vi "Testing.vi"() -> ()   [LabVIEW 2024]
uses:
  <vilib>/Instr/_visa.llb/VISA Configure Serial Port (Instr).vi
panel:
  out "FrequencyCounter":refnum<visa-resource-name>
  out "connection information":path
  in  "Database Checker":bool
  in  "Test Type":u16(ring)=1 items=["FVT/OSC/PHN", "FVT/OSC", "FVT/PHN", "OSC/PHN", "FVT", "OSC", "PHN", "Warmup", "Output Powers", "Warmup/Output Powers"]
  out "TITLE":string
  out "System Number":string
  in  "Functional Test":bool
  out "Functional Test Data":string
  out "Time":string
  out "System Status":string
  in  "Run Test(s)":bool
  in  "Exit":bool
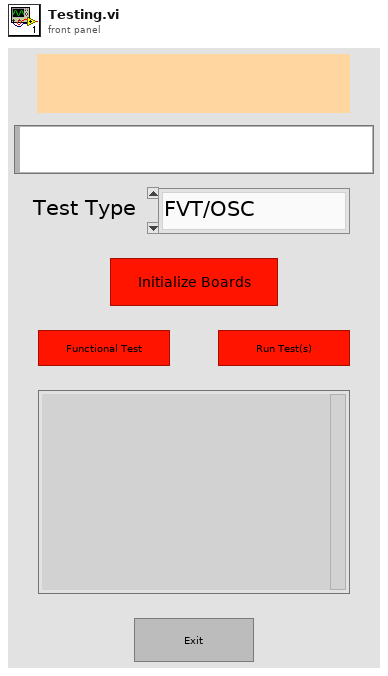
[diagram p1: front panel]
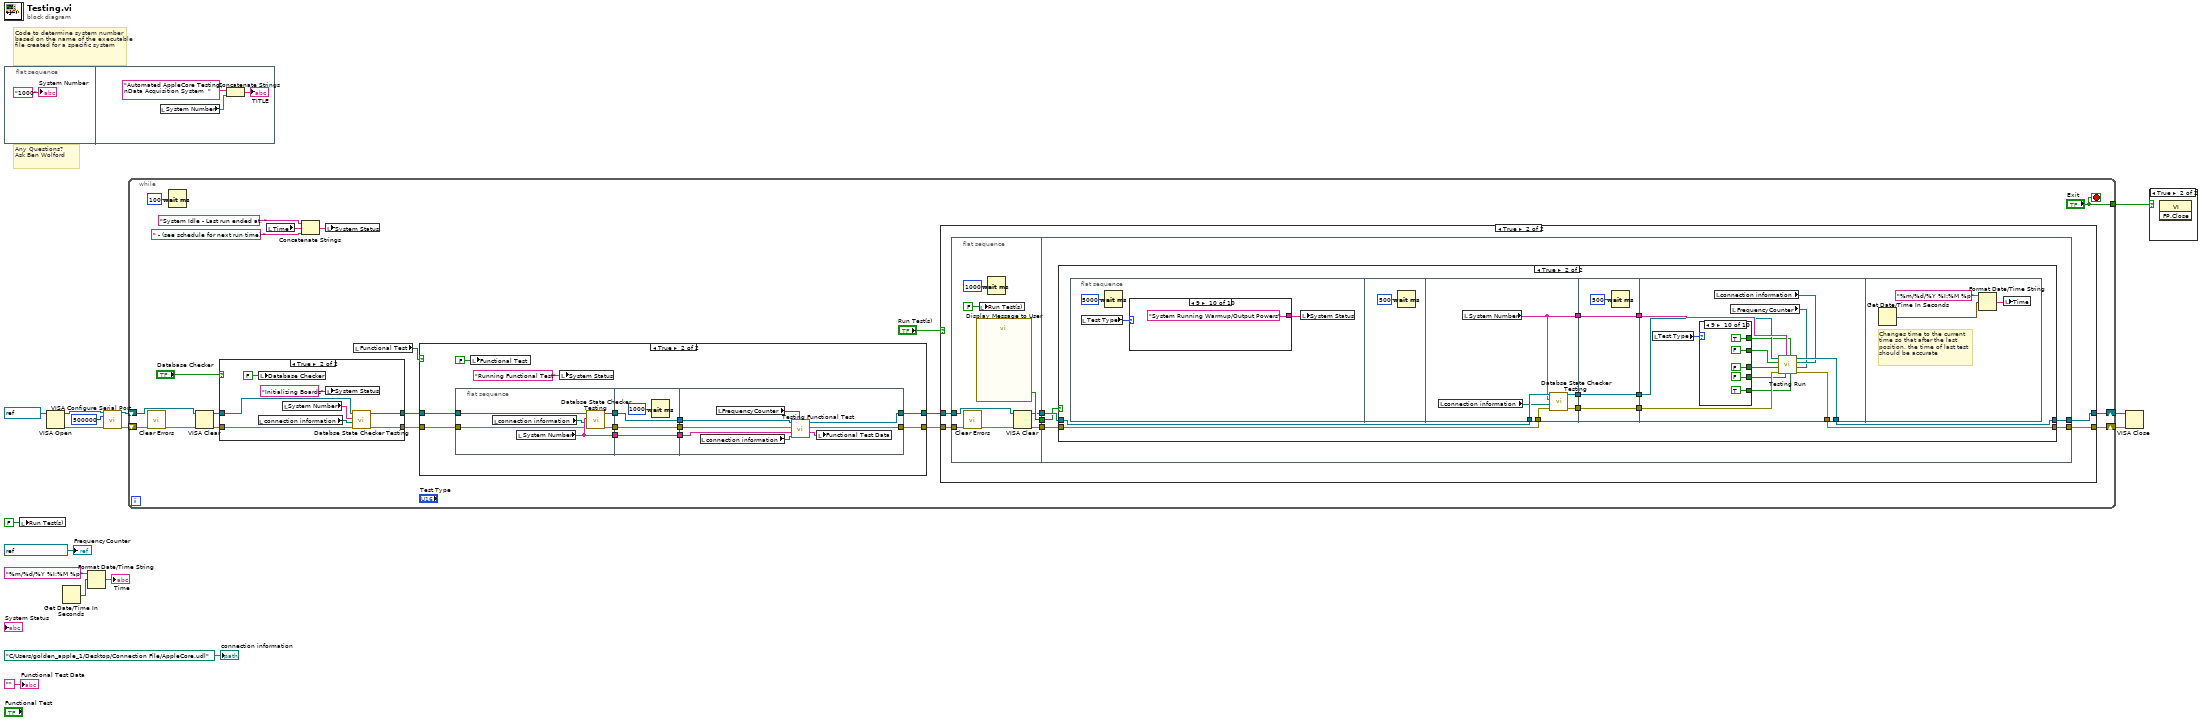
[diagram p0: block diagram]
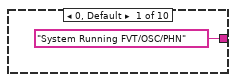
[diagram p7: hidden frame]
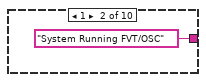
[diagram p8: hidden frame]
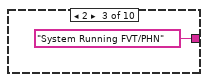
[diagram p9: hidden frame]
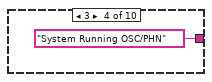
[diagram p10: hidden frame]
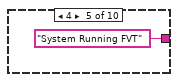
[diagram p11: hidden frame]
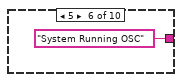
[diagram p12: hidden frame]
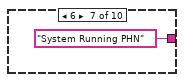
[diagram p13: hidden frame]
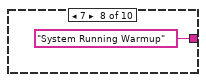
[diagram p14: hidden frame]
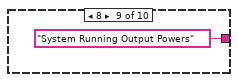
[diagram p15: hidden frame]
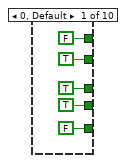
[diagram p16: hidden frame]
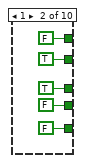
[diagram p17: hidden frame]
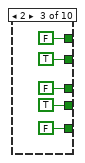
[diagram p18: hidden frame]
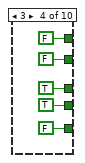
[diagram p19: hidden frame]
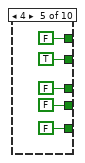
[diagram p20: hidden frame]
diagram:
  # "Any Questions?\nAsk Ben Wolford"
  # "Code to determine system number based on the name of the executable file created for a specific system"
  n1 = flat-sequence {
    frame #0 {
      "System Number" <- "1000" ("substring")
    }
    frame #1 {
      n2 = local read "System Number"() -> (w20:string)
      n3 = Concatenate Strings("Automated AppleCore Testing\nData Acquisition System  " ("TITLE"), w20) -> (→"TITLE":string)
    }
  }
  n4 = local write "Run Test(s)"(FALSE ("Run Test(s)")) -> ()
  n5 = VISA Open(VISA resource name=refnum<visa-resource-name> "COM4") -> (VISA resource name=w7:refnum<visa-resource-name>, error out=w6:errorcluster)  [unwired: 4 in]
  n6 = Get Date/Time In Seconds() -> (seconds since 1Jan1904=w15:timestamp)
  n7 = Format Date/Time String(time format string (%c)="%m/%d/%Y %I:%M %p", seconds (now)=w15) -> (date/time string=→"Time":string)  [unwired: 1 in]
  n8 = call-poly "VISA Configure Serial Port"("VISA resource name"=w7, "baud rate (9600)"=u32 500000, "error in (no error)"=w6) -> ("VISA resource name out"=w5:refnum<visa-resource-name>, "error out"=w4:errorcluster)  [unwired: 11 in]
  n9 = while {
    shift-right: [w39] -> w9
    shift-left: w4 -> [w31]
    shift-right: [w38] -> w8
    shift-left: w5 -> [w33]
    tunnel: ["Exit"] -> w11
    stop <- "Exit" stop-if-true
    n10 = call <vilib>:"Clear Errors.vi"("error in (no error)"=w31) -> ("error out"=w32:errorcluster)  [unwired: 5 in, 1 out]
    n11 = Wait (ms)(milliseconds to wait=u32 100) -> ()  [unwired: 1 out]
    n12 = VISA Clear(VISA resource name=w33, error in (no error)=w32) -> (VISA resource name out=w25:refnum<visa-resource-name>, error out=w23:errorcluster)
    n13 = case shown="True" "Database Checker" {
      tunnel: w25 -> [w42 w50]
      tunnel: [w42 w49] -> w24
      tunnel: w23 -> [w41 w48]
      tunnel: [w41 w47] -> w22
      frame False {
      }
      frame True {
        n14 = local read "connection information"() -> (w43:path)
        n15 = local write "Database Checker"(FALSE ("Database Checker")) -> ()
        n16 = local read "System Number"() -> (w46:string)
        n17 = local write "System Status"("Initializing Boards") -> ()
        n18 = call "Databse State Checker Testing.vi"("error in"=w48, "connection information"=w43, "System Number"=w46, "Arduino"=w50) -> ("error out"=w47:errorcluster, "Arduino out"=w49:refnum<visa-resource-name>)  [unwired: 6 in]
      }
    }
    n19 = local read "Time"() -> (w30:string)
    n20 = Concatenate Strings("System Idle - Last run ended at: " ("System Status"), w30, " - (see schedule for next run time) " ("System Status")) -> (w29:string)
    n21 = local write "System Status"(w29) -> ()
    n22 = local read "Functional Test"() -> (w34:bool)
    n23 = case shown="True" w34 {
      tunnel: w24 -> [w52 w63]
      tunnel: [w52 w60] -> w36
      tunnel: [w51 w61] -> w37
      tunnel: w22 -> [w51 w62]
      frame False {
      }
      frame True {
        n24 = flat-sequence {
          tunnel: w63 -> [w68]
          tunnel: w62 -> [w66]
          tunnel: [w70] -> w59
          tunnel: [w69] -> w57
          tunnel: [w67] -> w55
          tunnel: w59 -> [w74]
          tunnel: [w74] -> w58
          tunnel: w57 -> [w73]
          tunnel: [w73] -> w56
          tunnel: w55 -> [w72]
          tunnel: [w72] -> w54
          tunnel: w58 -> [w80]
          tunnel: w56 -> [w79]
          tunnel: w54 -> [w81]
          tunnel: [w78] -> w61
          tunnel: [w77] -> w60
          frame #0 {
            n25 = local read "connection information"() -> (w65:path)
            n26 = local read "System Number"() -> (w67:string)
            n27 = call "Databse State Checker Testing.vi"("error in"=w66, "connection information"=w65, "System Number"=w67, "Arduino"=w68) -> ("error out"=w70:errorcluster, "Arduino out"=w69:refnum<visa-resource-name>)  [unwired: 6 in]
          }
          frame #1 {
            n28 = Wait (ms)(milliseconds to wait=u32 1000) -> ()  [unwired: 1 out]
          }
          frame #2 {
            n29 = local read "connection information"() -> (w76:path)
            n30 = local read "FrequencyCounter"() -> (w75:refnum<visa-resource-name>)
            n31 = call "Testing Functional Test.vi"("FrequencyCounter"=w75, "connection information"=w76, "System Number"=w81, "error in"=w80, "Arduino"=w79) -> ("Functional Test Data"=w82:string, "error out"=w78:errorcluster, "Arduino"=w77:refnum<visa-resource-name>)  [unwired: 4 in]
            n32 = local write "Functional Test Data"(w82) -> ()
          }
        }
        n33 = local write "Functional Test"(FALSE ("Functional Test")) -> ()
        n34 = local write "System Status"("Running Functional Test") -> ()
      }
    }
    n35 = case shown="True" "Run Test(s)" {
      tunnel: w37 -> [w83 w88]
      tunnel: w36 -> [w84 w87]
      tunnel: [w83 w86] -> w39
      tunnel: [w84 w85] -> w38
      frame False {
      }
      frame True {
        n36 = flat-sequence {
          tunnel: [w99] -> w91
          tunnel: [w97] -> w90
          tunnel: [w96] -> w89
          tunnel: w87 -> [w93]
          tunnel: w88 -> [w94]
          tunnel: [w103] -> w86
          tunnel: [w104] -> w85
          tunnel: w89 -> [w102]
          tunnel: w90 -> [w101]
          tunnel: w91 -> [w100]
          frame #0 {
            n37 = call <vilib>:"Clear Errors.vi"("error in (no error)"=w94) -> ("error out"=w95:errorcluster)  [unwired: 5 in, 1 out]
            n38 = call "Display Message to User"() -> ("Yes"=w99:bool)  [unwired: 10 in, 1 out]
            n39 = local write "Run Test(s)"(FALSE ("Force Readings\nNOW!")) -> ()
            n40 = Wait (ms)(milliseconds to wait=u32 1000) -> ()  [unwired: 1 out]
            n41 = VISA Clear(VISA resource name=w93, error in (no error)=w95) -> (VISA resource name out=w97:refnum<visa-resource-name>, error out=w96:errorcluster)
          }
          frame #1 {
            n42 = case shown="True" w100 {
              tunnel: w101 -> [w106 w114]
              tunnel: w102 -> [w105 w113]
              tunnel: [w106 w116] -> w104
              tunnel: [w105 w115] -> w103
              frame False {
              }
              frame True {
                n43 = flat-sequence {
                  tunnel: w114 -> [w136]
                  tunnel: w113 -> [w135]
                  tunnel: [w132] -> w112
                  tunnel: [w134] -> w110
                  tunnel: [w133] -> w108
                  tunnel: w112 -> [w140]
                  tunnel: [w140] -> w111
                  tunnel: w110 -> [w139]
                  tunnel: [w139] -> w109
                  tunnel: w108 -> [w138]
                  tunnel: [w138] -> w107
                  tunnel: [w152] -> w116
                  tunnel: [w153] -> w115
                  tunnel: w111 -> [w149]
                  tunnel: w109 -> [w148]
                  tunnel: w107 -> [w147]
                  frame #0 {
                    n44 = local read "Test Type"() -> (w118:u16)
                    n45 = Wait (ms)(milliseconds to wait=u32 5000) -> ()  [unwired: 1 out]
                    n46 = case shown="9" w118 {
                      tunnel: ["System Running FVT/OSC/PHN" ("System Status") "System Running FVT/OSC" ("System Status") "System Running FVT/PHN" ("System Status") "System Running OSC/PHN" ("System Status") "System Running FVT" ("System Status") "System Running OSC" ("System Status") "System Running PHN" ("System Status") "System Running Warmup" ("System Status") "System Running Output Powers" ("System Status") "System Running Warmup/Output Powers" ("System Status")] -> w117
                      frame 0, Default {
                      }
                      frame 1 {
                      }
                      frame 2 {
                      }
                      frame 3 {
                      }
                      frame 4 {
                      }
                      frame 5 {
                      }
                      frame 6 {
                      }
                      frame 7 {
                      }
                      frame 8 {
                      }
                      frame 9 {
                      }
                    }
                    n47 = local write "System Status"(w117) -> ()
                  }
                  frame #1 {
                    n48 = Wait (ms)(milliseconds to wait=u32 500) -> ()  [unwired: 1 out]
                  }
                  frame #2 {
                    n49 = local read "connection information"() -> (w131:path)
                    n50 = local read "System Number"() -> (w132:string)
                    n51 = call "Databse State Checker Testing.vi"("error in"=w135, "connection information"=w131, "System Number"=w132, "Arduino"=w136) -> ("error out"=w133:errorcluster, "Arduino out"=w134:refnum<visa-resource-name>)  [unwired: 6 in]
                  }
                  frame #3 {
                    n52 = Wait (ms)(milliseconds to wait=u32 500) -> ()  [unwired: 1 out]
                  }
                  frame #4 {
                    n53 = local read "Test Type"() -> (w146:u16)
                    n54 = case shown="9" w146 {
                      tunnel: [TRUE TRUE TRUE FALSE TRUE FALSE FALSE FALSE FALSE FALSE] -> w150
                      tunnel: [TRUE TRUE FALSE TRUE FALSE TRUE FALSE FALSE FALSE FALSE] -> w151
                      tunnel: [TRUE FALSE TRUE TRUE FALSE FALSE TRUE FALSE FALSE FALSE] -> w145
                      tunnel: [FALSE FALSE FALSE FALSE FALSE FALSE FALSE FALSE TRUE TRUE] -> w144
                      tunnel: [FALSE FALSE FALSE FALSE FALSE FALSE FALSE TRUE FALSE TRUE] -> w143
                      frame 0, Default {
                      }
                      frame 1 {
                      }
                      frame 2 {
                      }
                      frame 3 {
                      }
                      frame 4 {
                      }
                      frame 5 {
                      }
                      frame 6 {
                      }
                      frame 7 {
                      }
                      frame 8 {
                      }
                      frame 9 {
                      }
                    }
                    n55 = local read "connection information"() -> (w142:path)
                    n56 = local read "FrequencyCounter"() -> (w141:refnum<visa-resource-name>)
                    n57 = call "Testing Run.vi"("FrequencyCounter"=w141, "connection information"=w142, "Output Powers"=w144, "Warmup"=w143, "PHN Test"=w145, "System Number"=w149, "error in"=w147, "Osc Test"=w151, "FVT Test"=w150, "Arduino"=w148) -> ("error out"=w153:errorcluster, "Arduino out"=w152:refnum<visa-resource-name>)
                  }
                  frame #5 {
                    # "Changes time to the current time so that after the last position, the time of last test should be accurate"
                    n58 = Get Date/Time In Seconds() -> (seconds since 1Jan1904=w205:timestamp)
                    n59 = Format Date/Time String(time format string (%c)="%m/%d/%Y %I:%M %p", seconds (now)=w205) -> (date/time string=w206:string)  [unwired: 1 in]
                    n60 = local write "Time"(w206) -> ()
                  }
                }
              }
            }
          }
        }
      }
    }
  }
  n61 = VISA Close(VISA resource name=w8, error in (no error)=w9) -> ()  [unwired: 1 out]
  n62 = case shown="True" w11 {
    frame False {
    }
    frame True {
      n63 = invoke class="VI" method="FP.Close"() -> ()  [unwired: 3 in, 3 out]
    }
  }
  "Functional Test Data" <- ""
  "connection information" <- path "C:/Users/golden_apple_1/Desktop/Connection File/AppleCore.udl" ("connection information")
  "FrequencyCounter" <- refnum<visa-resource-name> "GPIB0::3::INSTR" ("FrequencyCounter")
